vi "add_line_to_enface.vi"(0 "En Face Image":T1, 1 "Shift":i32=1, 5 "Raw Image":T1, 7 "Add Height":dbl=1.0, 9 "Input Line":i32=1, 11 "error in (no error)":errorcluster, 12 "Output Line":dbl) -> (4 "En Face Image Out":T1, 15 "error out":errorcluster)   [LabVIEW 2016]
doc: "Adds the next line to the en face or fluorescence image. The raw images can either be an OCT B-scan, in which case a single depth line (T scan) is extracted or a fluorescence line, in which case 'input line must be set to zero. If we have moved more then one line in the output image then the input line is simply copied multiple times to fill the space (zero order interpolation)"
uses:
  <vilib>/vision/Image Controls.llb/IMAQ Image.ctl
  <vilib>/vision/NI_Vision_Development_Module.lvlib
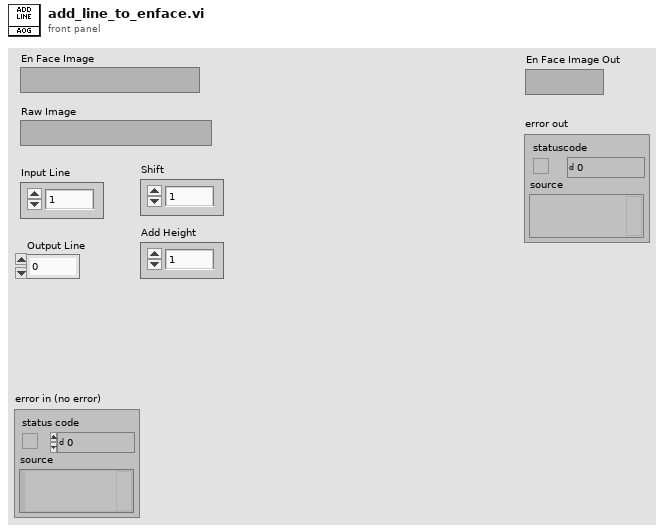
[diagram p1: front panel]
types:
  T1 = typedef "IMAQ Image.ctl" = refnum<image>
  T2 = typedef "Image Type" = u32
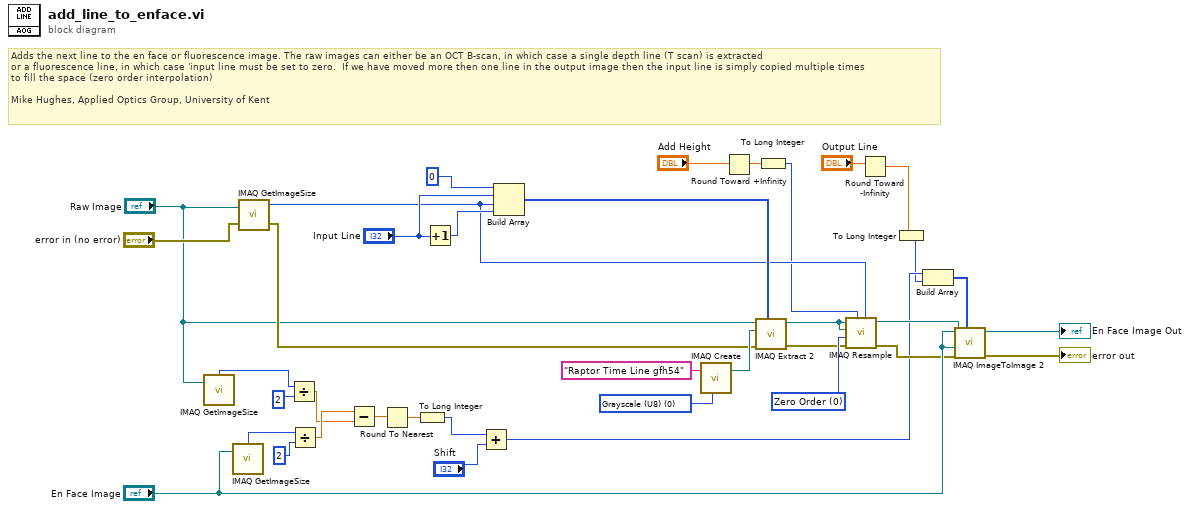
[diagram p0: block diagram]
diagram:
  w15 = u32 0 items=["Zero Order", "Bi-Linear", "Quadratic", "Cubic Spline"] ("Interpolation Type")
  w35 = T2 0 items=["Grayscale (U8)", "Grayscale (I16)", "Grayscale (SGL)", "Complex (CSG)", "RGB (U32)", "HSL (U32)", "RGB (U64)", "Grayscale (U16)"] ("Image Type")
  # "Adds the next line to the en face or fluorescence image. The raw images can either be an OCT B-scan, in which case a single depth line (T scan) is extracted\nor a fluorescence line, in which case 'input line must be set to zero.  If we have moved more then one line in the output image then the input line is simply copied multiple times\nto fill the space (zero order interpolation)\n\nMike Hughes, Applied Optics Group, University of Kent"
  n1 = call "IMAQ GetImageSize"("Image"="Raw Image") -> ("X Resolution"=w20:i32)  [unwired: 3 in, 2 out]
  n2 = call "IMAQ GetImageSize"("Image"="En Face Image") -> ("X Resolution"=w24:i32)  [unwired: 3 in, 2 out]
  n3 = call "IMAQ GetImageSize"("Image"="Raw Image", "error in (no error)"="error in (no error)") -> ("X Resolution"=w14:i32, "error out"=w28:errorcluster)  [unwired: 2 in, 1 out]
  n4 = Divide(x=w20, y=2) -> (x/y=w18:dbl)
  n5 = Divide(x=w24, y=2) -> (x/y=w19:dbl)
  n6 = Subtract(x=w19, y=w18) -> (x-y=w6:dbl)
  n7 = Round To Nearest(number=w6) -> (nearest integer value=w5:dbl)
  n8 = To Long Integer(number=w5) -> (32bit integer=w4:i32)
  n9 = Increment(x="Input Line") -> (x+1=w26:i32)
  n10 = Add(x=w4, y="Shift") -> (x+y=w3:i32)
  n11 = Build Array(0 ("element"), "Input Line", w14, w26) -> (w33:i32[])
  n12 = call "IMAQ Create"("Image Name"="Raptor Time Line gfh54", "Image Type"=w35) -> ("New Image"=w34:T1)  [unwired: 3 in, 1 out]
  n13 = Round Toward +Infinity(x="Add Height") -> (ceil(x): smallest int >= x=w8:dbl)
  n14 = call "IMAQ Extract 2"("Optional Rectangle"=w33, "error in (no error)"=w28, "Image Dst"=w34, "Image Src"="Raw Image") -> ("error out"=w11:errorcluster, "Image Dst Out"=w16:T1)  [unwired: 6 in]
  n15 = To Long Integer(number=w8) -> (32bit integer=w7:i32)
  n16 = call "IMAQ Resample"("X Resolution"=w14, "Y Resolution"=w7, "error in (no error)"=w11, "Interpolation Type"=w15, "Image Dst"=w16, "Image Src"=w16) -> ("error out"=w12:errorcluster, "Image Dst Out"=w13:T1)  [unwired: 4 in]
  n17 = Round Toward -Infinity(1:"Output Line") -> (0:w2:dbl)
  n18 = To Long Integer(number=w2) -> (32bit integer=w1:i32)
  n19 = Build Array(w3, w1) -> (w32:i32[])
  n20 = call "IMAQ ImageToImage 2"("Offset Left/Top"=w32, "error in (no error)"=w12, "Image Dst"="En Face Image", "Image Src (Small)"=w13, "Image Src (Large)"="En Face Image") -> ("error out"=→"error out":errorcluster, "Image Dst Out"=→"En Face Image Out":T1)  [unwired: 5 in]
